vi "Read.vi"(8 "error in":errorcluster, 11 "Device Cluster.lvclass in":refnum<class "Device Cluster.lvclass">) -> (0 "error out":errorcluster, 3 "Device Cluster.lvclass out":refnum<class "Device Cluster.lvclass">)   [LabVIEW 2023, in "Device Cluster.lvclass"]
uses:
  Device Cluster.lvclass
  Device Cluster.lvclass/Device Cluster.ctl
  79148ede-8dcf-4e1a-92ea-577e44e144f7.vi
  36a813f2-0d4e-4d87-b43e-db3b43b61d5e.vi
  79148ede-8dcf-4e1a-92ea-577e44e144f7.vi/c28b0ead-42ad-4072-80a2-aca7f2bd7ce3.vi
  79148ede-8dcf-4e1a-92ea-577e44e144f7.vi/219d0231-d98b-4193-b5cc-84f90e3c9091.vi
  36a813f2-0d4e-4d87-b43e-db3b43b61d5e.vi/c28b0ead-42ad-4072-80a2-aca7f2bd7ce3.vi
  36a813f2-0d4e-4d87-b43e-db3b43b61d5e.vi/219d0231-d98b-4193-b5cc-84f90e3c9091.vi
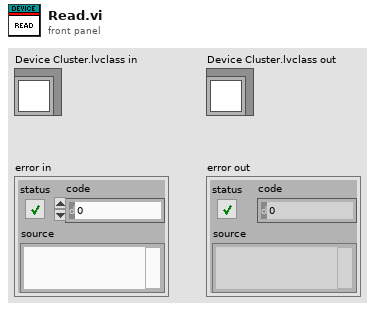
[diagram p1: front panel]
types:
  T1 = typedef "Cluster.lvclass/Consumer Control.ctl" = cluster{"OnOff.ACT":bool, "ErrorAcknowledge.ACT":bool}
  T2 = typedef "Cluster.lvclass/Consumer Ch.ctl" = cluster{"OutputEnable.ACT":bool, "ControlMode.CTL":u16, "Setpoint.SP":dbl}
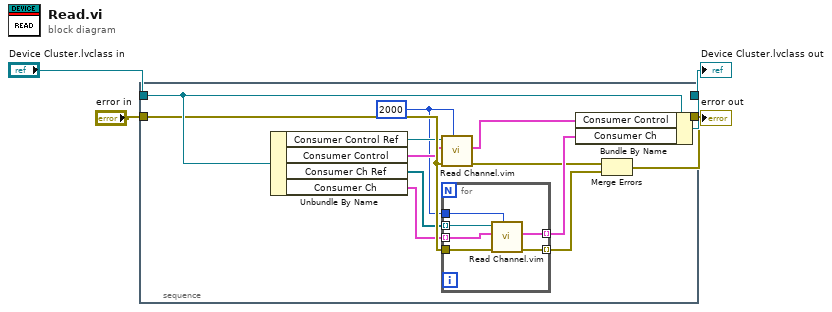
[diagram p0: block diagram]
diagram:
  n1 = stacked-sequence {
    tunnel: [w14] -> w4
    tunnel: [w15] -> w3
    tunnel: "error in" -> [w10]
    tunnel: "Device Cluster.lvclass in" -> [w11]
    frame #0 {
      w5 = 2000 ("Timeout (ms)")
      n2 = Unbundle By Name(w11) -> ("Consumer Control Ref"=w6:refnum<k21>, "Consumer Control"=w7:T1, "Consumer Ch Ref"=w8:refnum<k21>[], "Consumer Ch"=w9:T2[])
      n3 = call "Read Channel.vim"("Timeout (ms)"=w5, "error in"=w10, "Data in"=w7, "ADAS HIL Channel in"=w6) -> ("error out"=w13:errorcluster, "Data out"=w16:T1)  [unwired: 4 in, 2 out]
      n4 = for {
        tunnel: w5 -> [w23]
        tunnel: w8 -> [w22] mode=indexing
        tunnel: w9 -> [w21] mode=indexing
        tunnel: w10 -> [w20]
        tunnel: [w19] -> w17 mode=indexing
        tunnel: [w18] -> w12 mode=indexing
        n5 = call "Read Channel.vim"("Timeout (ms)"=w23, "error in"=w20, "Data in"=w21, "ADAS HIL Channel in"=w22) -> ("error out"=w18:errorcluster, "Data out"=w19:T2)  [unwired: 4 in, 2 out]
      }
      n6 = Bundle By Name(cluster=w11, "Consumer Control"=w16, "Consumer Ch"=w17) -> (w15:refnum<class "Device Cluster.lvclass">)
      n7 = Merge Errors(w13, w12) -> (w14:errorcluster)
    }
  }
  "error out" <- w4
  "Device Cluster.lvclass out" <- w3
